vi "Settings Box.vi"(8 "error in (no error)":errorcluster, 11 "Instrument array":refnum<class "Instrument.lvclass">[](array[class])) -> (0 "error out":errorcluster, 1 "statusbox":string, 3 "Instrument Array out":refnum<class "Instrument.lvclass">[](array[class]))   [LabVIEW 2009]
uses:
  Instruments/Utility Classes/Instrument/Instrument.lvclass
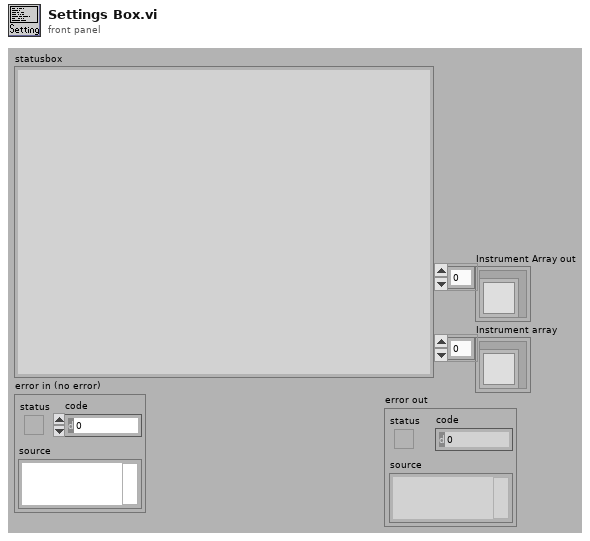
[diagram p1: front panel]
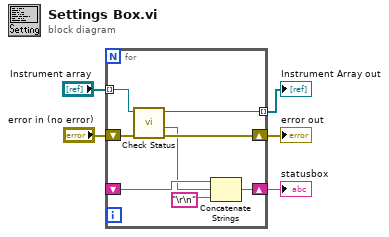
[diagram p0: block diagram]
diagram:
  n1 = for {
    tunnel: [w13] -> w5 mode=indexing
    tunnel: "Instrument array" -> [w12] mode=indexing
    shift-right: [w10] -> w2
    shift-left: "error in (no error)" -> [w11]
    shift-right: [w8] -> w1
    shift-left: _ -> [w9]
    n2 = call-dynamic "Check Status.vi"("error in (no error)"=w11, "Instrument in"=w12) -> ("error out"=w10:errorcluster, "Status"=w7:string, "Instrument out"=w13:refnum<class "Instrument.lvclass">)  [unwired: 7 out]
    n3 = Concatenate Strings(w9, w7, "\r\n") -> (w8:string)
  }
  "statusbox" <- w1
  "Instrument Array out" <- w5
  "error out" <- w2
